vi "Get Multi.vi"(0 "Display State In":T2, 5 "Value In":T1={"Active"=FALSE, "Delay (ms)"=0.0, "Duration (ms)"=50.0, "Ramp (ms)"=5.0, "Rate (Hz)"=0.0, "Trepeat (ms)"=0.0, "Repeat"=FALSE}, 9 "Container State":T3, 11 "error in (no error)":errorcluster) -> (4 "Display State Out":T2, 6 "Value Out":T1={"Active"=FALSE, "Delay (ms)"=0.0, "Duration (ms)"=50.0, "Ramp (ms)"=5.0, "Rate (Hz)"=0.0, "Trepeat (ms)"=0.0, "Repeat"=FALSE}, 15 "error out":errorcluster)   [LabVIEW 2015, in "Burst (G3).xctl"]
uses:
  Burst (G3).xctl
  <vilib>/_xctls/Container State.ctl
  State.ctl
  Utility VIs/Controls/KCheckbox/KCheckbox.xctl
  Utility VIs/Controls/KNumeric (DBL)/KNumeric (DBL).xctl
  Burst Data.ctl
  <vilib>/_xctls/XControlSupport.lvlib
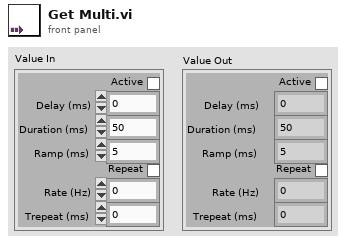
[diagram p1: front panel]
types:
  T1 = typedef "Burst (G3).xctl/Burst Data.ctl" = cluster{"Active":bool, "Delay (ms)":dbl, "Duration (ms)":dbl, "Ramp (ms)":dbl, "Rate (Hz)":dbl, "Trepeat (ms)":dbl, "Repeat":bool}
  T2 = typedef "Burst (G3).xctl/State.ctl" = cluster{"ctls":cluster{"Active":refnum<vi>, "Delay":refnum<vi>, "Dur":refnum<vi>, "Ramp":refnum<vi>, "Repeat":refnum<vi>, "at":refnum<vi>, "for":refnum<vi>}, "active mixed":bool, "repeat mixed":bool}
  T3 = typedef "XControlSupport.lvlib/Container State.ctl" = cluster{"Indicator?":bool, "Run Mode?":bool, " Refnum":refnum<vi>}
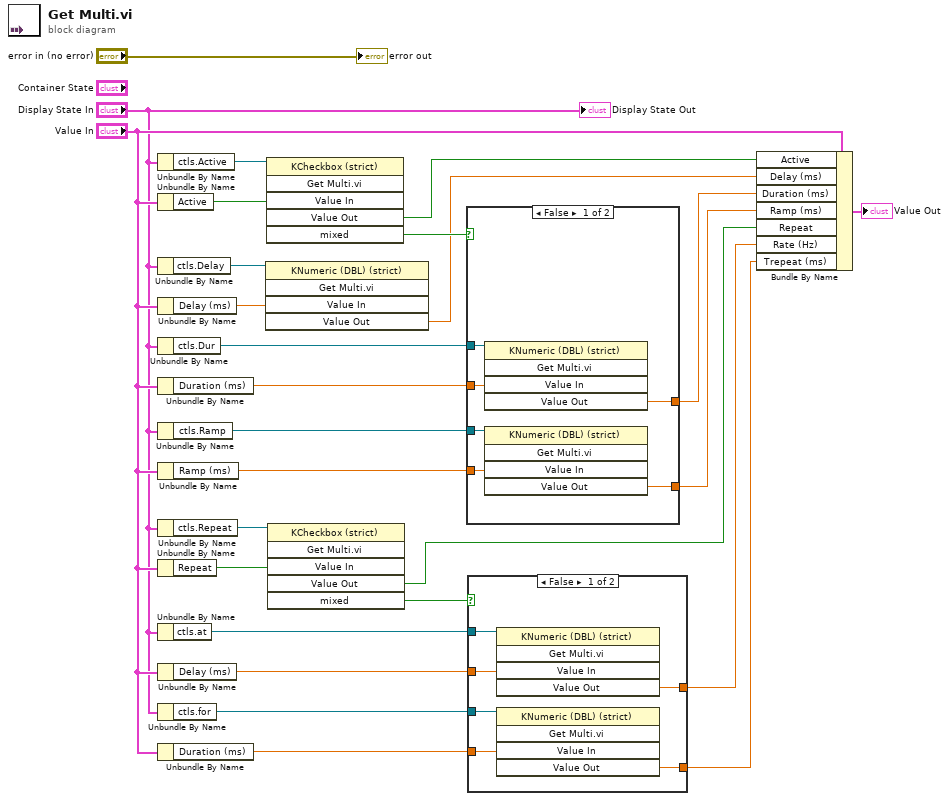
[diagram p0: block diagram]
diagram:
  n1 = Unbundle By Name("Display State In") -> ("ctls.Active"=w26:refnum<vi>)
  n2 = Unbundle By Name("Value In") -> ("Active"=w25:bool)
  n3 = Unbundle By Name("Display State In") -> ("ctls.Delay"=w3:refnum<vi>)
  n4 = Unbundle By Name("Value In") -> ("Delay (ms)"=w2:dbl)
  n5 = Unbundle By Name("Display State In") -> ("ctls.Dur"=w23:refnum<vi>)
  n6 = Unbundle By Name("Value In") -> ("Duration (ms)"=w22:dbl)
  n7 = Unbundle By Name("Display State In") -> ("ctls.Ramp"=w21:refnum<vi>)
  n8 = Unbundle By Name("Value In") -> ("Ramp (ms)"=w20:dbl)
  n9 = Unbundle By Name("Display State In") -> ("ctls.Repeat"=w16:refnum<vi>)
  n10 = Unbundle By Name("Value In") -> ("Repeat"=w15:bool)
  n11 = Unbundle By Name("Display State In") -> ("ctls.at"=w11:refnum<vi>)
  n12 = Unbundle By Name("Value In") -> ("Delay (ms)"=w9:dbl)
  n13 = Unbundle By Name("Display State In") -> ("ctls.for"=w10:refnum<vi>)
  n14 = Unbundle By Name("Value In") -> ("Duration (ms)"=w8:dbl)
  n15 = invoke class="KNumeric (DBL) (strict)" method="Get Multi.vi"(reference=w3, "Value In"=w2) -> ("Value Out"=w1:dbl)  [unwired: 3 in, 4 out]
  n16 = invoke class="KCheckbox (strict)" method="Get Multi.vi"(reference=w26, "Value In"=w25) -> ("Value Out"=w24:bool, "mixed"=w19:bool)  [unwired: 4 in, 4 out]
  n17 = invoke class="KCheckbox (strict)" method="Get Multi.vi"(reference=w16, "Value In"=w15) -> ("Value Out"=w7:bool, "mixed"=w14:bool)  [unwired: 4 in, 4 out]
  n18 = case shown="False" w19 {
    tunnel: w23 -> [w33 _]
    tunnel: w22 -> [w32 w35]
    tunnel: w21 -> [w31 _]
    tunnel: w20 -> [w30 w34]
    tunnel: [w29 w35] -> w18
    tunnel: [w28 w34] -> w17
    frame False {
      n19 = invoke class="KNumeric (DBL) (strict)" method="Get Multi.vi"(reference=w33, "Value In"=w32) -> ("Value Out"=w29:dbl)  [unwired: 3 in, 4 out]
      n20 = invoke class="KNumeric (DBL) (strict)" method="Get Multi.vi"(reference=w31, "Value In"=w30) -> ("Value Out"=w28:dbl)  [unwired: 3 in, 4 out]
    }
    frame True {
    }
  }
  n21 = case shown="False" w14 {
    tunnel: w11 -> [w41 _]
    tunnel: w9 -> [w40 w43]
    tunnel: w10 -> [w39 _]
    tunnel: w8 -> [w38 w42]
    tunnel: [w37 w43] -> w6
    tunnel: [w36 w42] -> w5
    frame False {
      n22 = invoke class="KNumeric (DBL) (strict)" method="Get Multi.vi"(reference=w41, "Value In"=w40) -> ("Value Out"=w37:dbl)  [unwired: 3 in, 4 out]
      n23 = invoke class="KNumeric (DBL) (strict)" method="Get Multi.vi"(reference=w39, "Value In"=w38) -> ("Value Out"=w36:dbl)  [unwired: 3 in, 4 out]
    }
    frame True {
    }
  }
  n24 = Bundle By Name(cluster="Value In", "Active"=w24, "Delay (ms)"=w1, "Duration (ms)"=w18, "Ramp (ms)"=w17, "Repeat"=w7, "Rate (Hz)"=w6, "Trepeat (ms)"=w5) -> (→"Value Out":T1)
  "Display State Out" <- "Display State In"
  "error out" <- "error in (no error)"
